vi "Write_Open_File_int.vi"(0 "delimiter (Tab)":string="\t", 1 "transpose? (no:F)":bool, 4 "format (%.3f)":string="%.3f", 5 "error in":errorcluster, 6 "1D data":u32[](array[numeric]), 7 "2D data":u32[][](array[numeric]), 8 "refnum":refnum<file>) -> (3 "dup refnum":refnum<file>)   [LabVIEW 2018]
doc: "Converts a 2D or 1D array of single-precision numbers to a text string and writes the string to a new byte stream file or appends the string to an existing file."
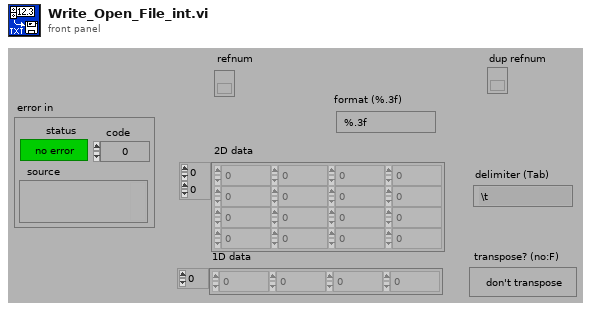
[diagram p1: front panel]
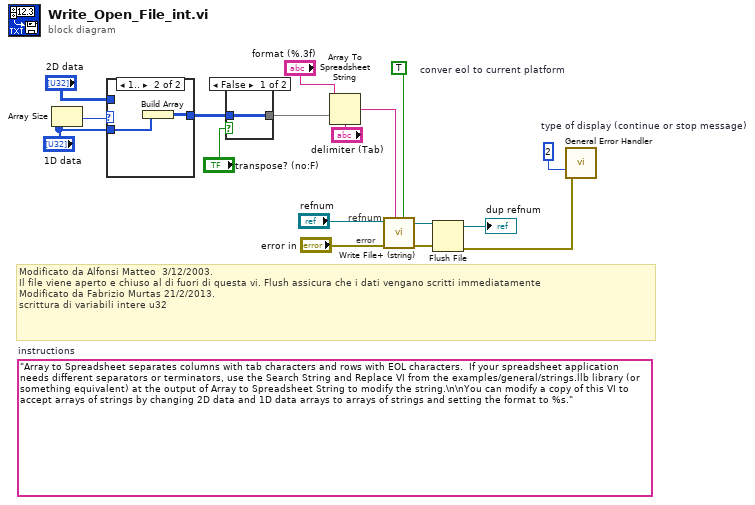
[diagram p0: block diagram]
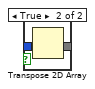
[diagram p2: hidden frame]
diagram:
  (unwired) "Array to Spreadsheet separates columns with tab characters and rows with EOL characters.  If your spreadsheet application needs different separators or terminators, use the Search String and Replace VI from the examples/general/strings.llb library (or something equivalent) at the output of Array to Spreadsheet String to modify the string.\n\nYou can modify a copy of this VI to accept arrays of strings by changing 2D data and 1D data arrays to arrays of strings and setting the format to %s."  # instructions
  w5 = TRUE  # conver eol to current platform
  w17 = 2  # type of display (continue or stop message)
  # "Modificato da Alfonsi Matteo  3/12/2003.\nIl file viene aperto e chiuso al di fuori di questa vi. Flush assicura che i dati vengano scritti immediatamente\nModificato da Fabrizio Murtas 21/2/2013.\nscrittura di variabili intere u32"
  # "error"
  # "refnum"
  n1 = Array Size(array="1D data") -> (size(s)=w15:i32)
  n2 = case shown="1.." w15 {
    tunnel: "1D data" -> [_ w20]
    tunnel: [w18 w19] -> w11
    tunnel: "2D data" -> [w18 _]
    frame ..0 {
      # "1D array is empty"
    }
    frame 1.. {
      n3 = Build Array(w20) -> (w19:u32[][])
    }
  }
  n4 = case shown="False" "transpose? (no:F)" {
    tunnel: [w21 w23] -> w9
    tunnel: w11 -> [w21 w22]
    frame False {
    }
    frame True {
      n5 = Transpose 2D Array(2D array=w22) -> (transposed array=w23:u32[][])
    }
  }
  n6 = Array To Spreadsheet String(delimiter (Tab)="delimiter (Tab)", array=w9, 3:"format (%.3f)") -> (spreadsheet string=w8:string)
  n7 = call <vilib>:"Write File+ (string).vi"("convert eol? (no:F)"=w5, "string"=w8, "error in (no error)"="error in", "refnum"="refnum") -> ("error out"=w16:errorcluster, "dup refnum"=w7:refnum<file>)  [unwired: 3 in, 1 out]
  n8 = Flush File(refnum=w7, error in=w16) -> (refnum out=→"dup refnum":refnum<file>, error out=w6:errorcluster)
  n9 = call <vilib>:"General Error Handler.vi"("type of dialog (OK msg:1)"=w17, "error in (no error)"=w6) -> ()  [unwired: 9 in, 5 out]
